vi "Open-FpgaNic.vi"   [LabVIEW 2017]
uses:
  Globals.vi
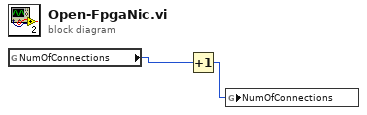
[diagram p0: block diagram]
diagram:
  n1 = global read "Globals.vi" "NumOfConnections"() -> (w1:u32)
  n2 = Increment(x=w1) -> (x+1=w2:u32)
  n3 = global write "Globals.vi" "NumOfConnections"(w2) -> ()
